vi "initialise.vi"(8 "error in (no error)":errorcluster, 11 "GenericPlugin in":refnum<class "GenericDAQ.lvclass">) -> (0 "error out":errorcluster, 3 "GenericPlugin out":refnum<class "GenericDAQ.lvclass">)   [LabVIEW 2010, in "GenericDAQ.lvclass"]
doc: "The dynamic dispatch-version of this VI initalises the plug-in object by allocating and initalising any dynamic resources need."
uses:
  GenericDAQ.lvclass
  common/classes/GenericToplevelComponent/GenericToplevelComponent/GenericToplevelComponent.lvclass
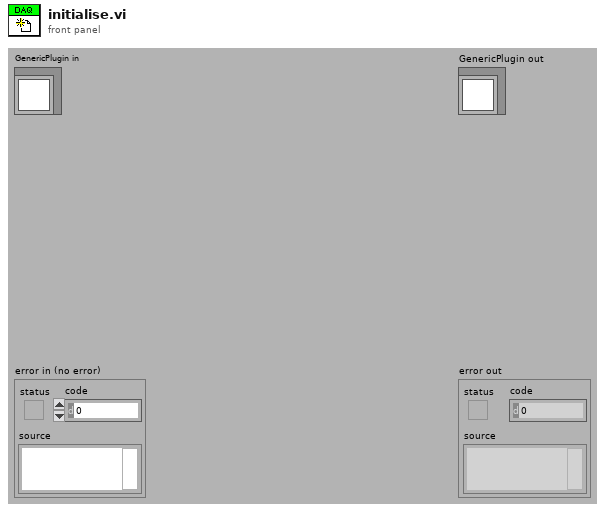
[diagram p1: front panel]
types:
  T1 = typedef "GenericToplevelComponent.lvclass/common_trigger_enum.ctl" = enum16{"NULL", "initialise", "terminate", "fetch command", "fetch data", "attach observer", "register as observer", "detach observer", "acknowledge", "start", "stop", "sweep started", "sweep finished", "experiment started", "experiment stopped"}
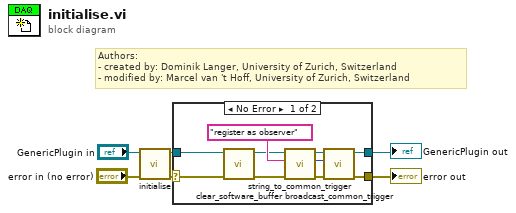
[diagram p0: block diagram]
diagram:
  # "Authors: \n- created by: Dominik Langer, University of Zurich, Switzerland\n- modified by: Marcel van 't Hoff, University of Zurich, Switzerland"
  n1 = call-parent "initialise.vi"("error in (no error)"="error in (no error)", "GenericPlugin in"="GenericPlugin in") -> ("error out"=w4:errorcluster, "GenericPlugin out"=w3:refnum<class "GenericDAQ.lvclass">)  [unwired: 8 in]
  n2 = case shown="No Error" w4 {
    selector: w4 -> [w14 w17]
    tunnel: w3 -> [w13 w18]
    tunnel: [w16 w17] -> w2
    tunnel: [w15 w18] -> w1
    frame No Error {
      n3 = call-dynamic "clear_software_buffer.vi"("error in (no error)"=w14, "GenericDAQ in"=w13) -> ("error out"=w12:errorcluster, "GenericDAQ out"=w8:refnum<class "GenericDAQ.lvclass">)  [unwired: 8 in]
      n4 = call-dynamic "string_to_common_trigger.vi"("error in (no error)"=w12, "trigger string"="register as observer" ("input string"), "GenericToplevelComponent in"=w8) -> ("error out"=w9:errorcluster, "trigger"=w10:T1, "GenericToplevelComponent out"=w7:refnum<class "GenericDAQ.lvclass">)  [unwired: 6 in]
      n5 = call-dynamic "broadcast_common_trigger.vi"("error in (no error)"=w9, "trigger"=w10, "GenericToplevelComponent in"=w7) -> ("error out"=w16:errorcluster, "GenericToplevelComponent out"=w15:refnum<class "GenericDAQ.lvclass">)  [unwired: 7 in]
    }
    frame Error {
    }
  }
  "error out" <- w2
  "GenericPlugin out" <- w1
